vi "TCPIP_test.vi"(5 "網路連線設定":cluster{"Address":string, "Port":u16}={"Address"="127.0.0.1", "Port"=8888} {"Port" min=1025 step=1}) -> (1 "String":string)   [LabVIEW 2020]
doc: "Displays data sent via TCP from Data Server.vi. Once a TCP connection is open, the VI reads 4 bytes to determine the amount of data being sent. It then reads and charts that many bytes. If an error occurs or the stop button is pressed, it sends a \"Q\" to the Data Sender to notify it to quit.\n\n<B>Note:</B> Requires the Data Server.vi located in the same library as this VI."
panel:
  in  "data in":string
  # "Instructions:\n1. Open the Data Server.vi located in the same library.\n2. Follow the instructions on it's front panel.\n\nNote: This VI is built to work with the Data Server.vi."
  # "數字(十進制顯示)"
  # "字串(假十進制)"
  # "check、input、button、stream\nFCT,1,192.168.132.70,input,SN_12345678\nFCT,1,192.168.132.70,button\nFCT,1,192.168.132.70,stream\nFCT,1,192.168.132.70,check"
  # "拆解字串(假十進制)"
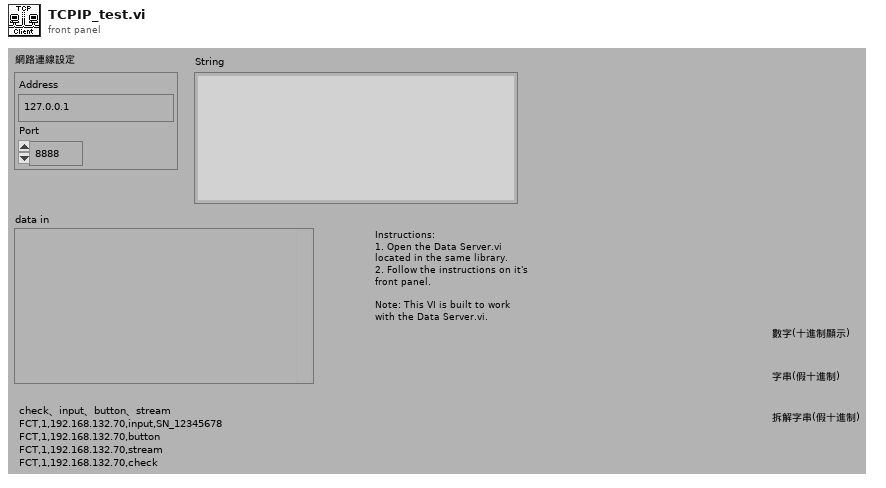
[diagram p1: front panel]
types:
  T1 = enum16{"Standard", "Buffered", "CRLF", "Immediate"}
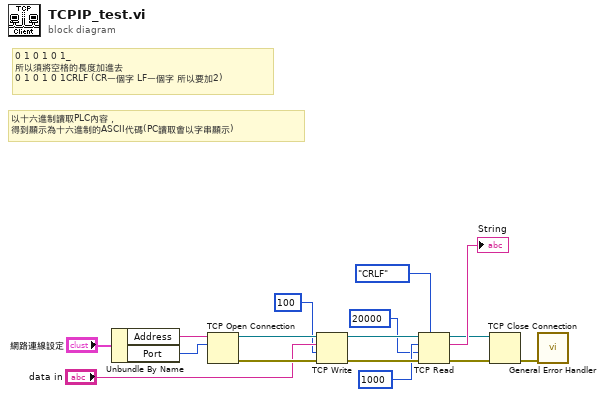
[diagram p0: block diagram]
diagram:
  # "0 1 0 1 0 1_\n所以須將空格的長度加進去\n0 1 0 1 0 1CRLF (CR一個字 LF一個字 所以要加2)"
  # "以十六進制讀取PLC內容，\n得到顯示為十六進制的ASCII代碼(PC讀取會以字串顯示)"
  n1 = Unbundle By Name("網路連線設定") -> ("Address"=w13:string, "Port"=w12:u16)
  n2 = TCP Open Connection(address=w13, remote port or service name=w12) -> (connection ID=w15:refnum<k5>, error out=w16:errorcluster)  [unwired: 1 in, 2 out]
  n3 = TCP Write(connection ID=w15, data in="data in", error in (no error)=w16, 9:100 ("timeout ms (25000)")) -> (connection ID out=w8:refnum<k5>, error out=w9:errorcluster)  [unwired: 1 out]
  n4 = TCP Read(connection ID=w8, bytes to read=1000, error in (no error)=w9, 7:T1."CRLF" ("mode (standard)"), 9:20000 ("timeout ms (25000)")) -> (connection ID out=w2:refnum<k5>, data out=→"String":string, error out=w1:errorcluster)
  n5 = TCP Close Connection(connection ID=w2, error in (no error)=w1) -> (error out=w10:errorcluster)  [unwired: 2 out]
  n6 = call <vilib>:"General Error Handler.vi"("error in (no error)"=w10) -> ()  [unwired: 2 in, 13 out]
